vi "updateSlaveStatus.vi"(8 "error in (no error)":errorcluster, 11 "camera status path 3":refnum<k21>) -> (1 "DeviceState":T1)   [LabVIEW 2018]
uses:
  support/State.ctl
  Tektronik3102/Tecktronik action loop.ctl
  CurrentSequenceStatus.vi
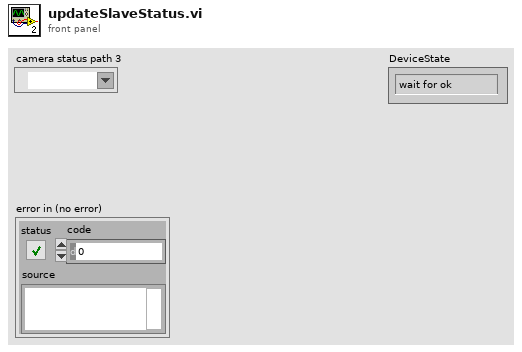
[diagram p1: front panel]
types:
  T1 = typedef "Tecktronik action loop.ctl" = enum16{"wait for ok", "error", "ready", "write log file", "waiting for connection", "exit", "sending command"}
  T2 = typedef "State.ctl" = cluster{"loop index":i32, "status":enum16{"busy", "ready", "error"}}
  T3 = cluster{"Camera done":bool, "Tektronik done":bool, "Motors done":bool}[]
  T4 = cluster{"Camera done":bool, "Tektronik done":bool, "Motors done":bool}
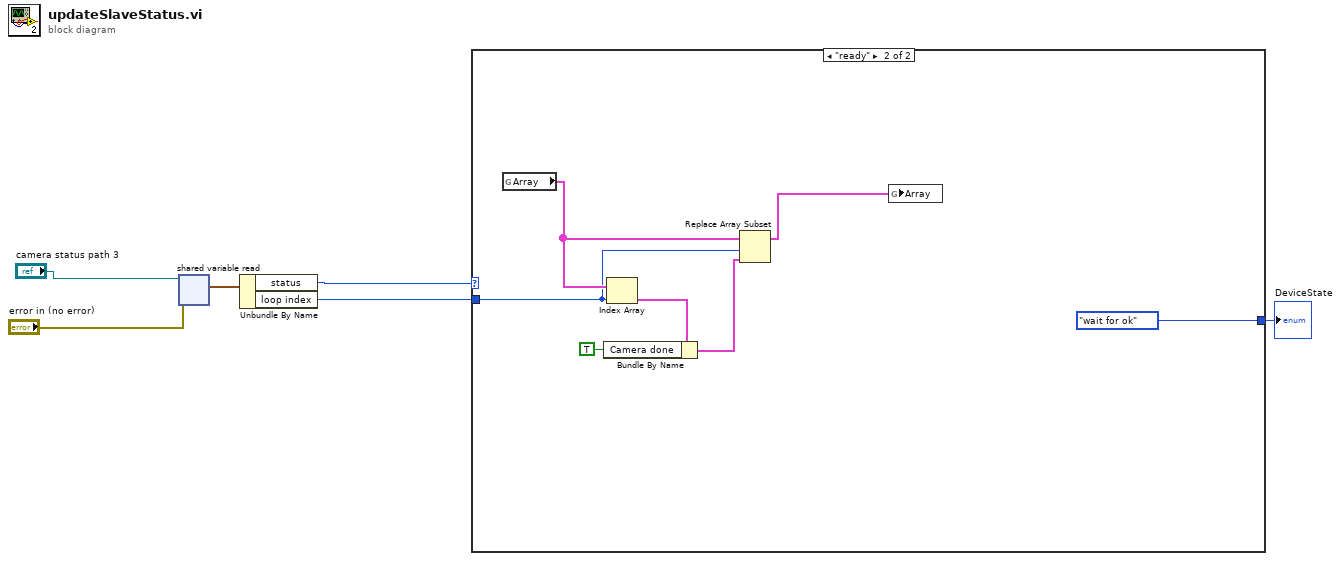
[diagram p0: block diagram]
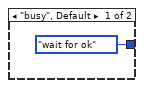
[diagram p2: hidden frame]
diagram:
  n1 = shared-variable-read("camera status path 3", "error in (no error)") -> (w6:T2)  [unwired: 3 out]
  n2 = Unbundle By Name(w6) -> ("status"=w3:enum16{"busy", "ready", "error"}, "loop index"=w2:i32)
  n3 = case shown="\"ready\"" w3 {
    tunnel: w2 -> [_ w13]
    tunnel: [Tecktronik_action_loop."wait for ok" ("DeviceState") Tecktronik_action_loop."wait for ok" ("DeviceState")] -> w1
    frame "busy", Default {
    }
    frame "ready" {
      n4 = global read "CurrentSequenceStatus.vi" "Array"() -> (w14:T3)
      n5 = Index Array(array=w14, index=w13) -> (element=w12:T4)
      n6 = Bundle By Name(cluster=w12, "Camera done"=TRUE) -> (w10:T4)
      n7 = Replace Array Subset(array=w14, new element=w10, index=w13) -> (w9:T3)
      n8 = global write "CurrentSequenceStatus.vi" "Array"(w9) -> ()
    }
  }
  "DeviceState" <- w1
